vi "Receive-and-verify.vi"(8 "error in (no error)":errorcluster, 9 "Match exactly?":bool, 10 "Expected return string":string, 11 "SM1000-control in":refnum<class "MC-SM1000.lvclass">) -> (0 "error out":errorcluster, 1 "Verified?":bool, 2 "Return string":string, 3 "SM1000-control out":refnum<class "MC-SM1000.lvclass">)   [LabVIEW 2013, in "MaterialCharacterization.lvlib" / "MC-SM1000.lvclass"]
doc: "Verified if the return string contains at least the \nexpected string. Case insensitive."
uses:
  MC-SM1000.lvclass
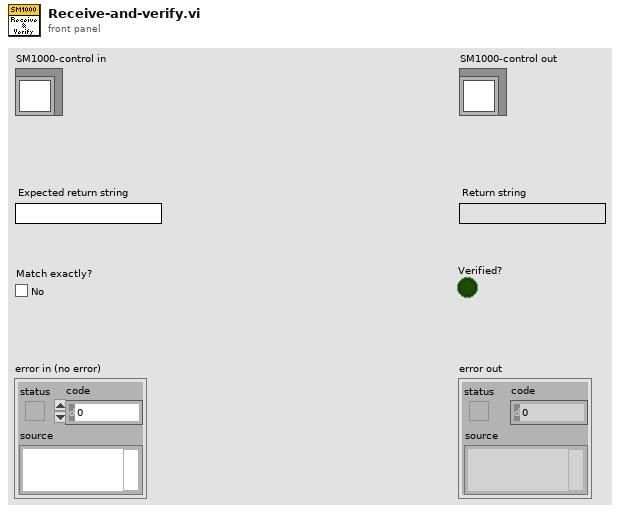
[diagram p1: front panel]
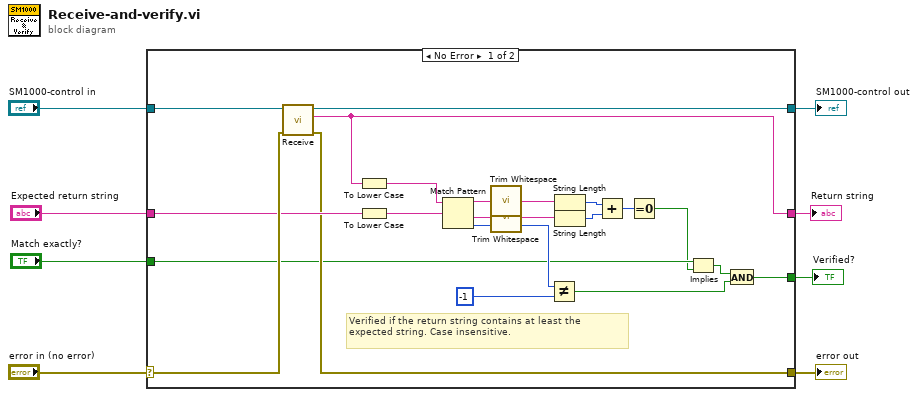
[diagram p0: block diagram]
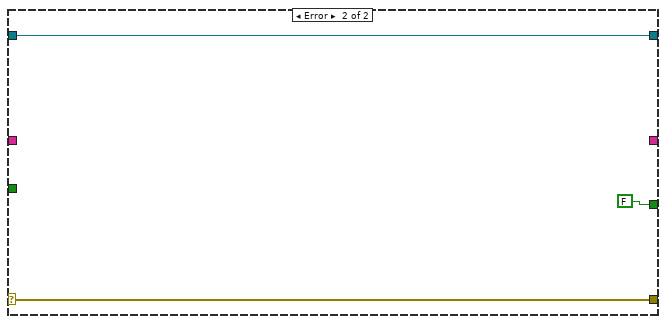
[diagram p2: hidden frame]
diagram:
  n1 = case shown="No Error" "error in (no error)" {
    selector: "error in (no error)" -> [w28 w33]
    tunnel: [w23 w33] -> w7
    tunnel: [w29 w32] -> w5
    tunnel: "SM1000-control in" -> [w30 w32]
    tunnel: [w24 _] -> w4
    tunnel: "Expected return string" -> [w27 _]
    tunnel: [w13 FALSE] -> w2
    tunnel: "Match exactly?" -> [w17 _]
    frame No Error {
      # "Verified if the return string contains at least the \nexpected string. Case insensitive."
      n2 = call "Receive.vi"("error in (no error)"=w28, "SM1000-control in"=w30) -> ("error out"=w23:errorcluster, "Return string"=w24:string, "SM1000-control out"=w29:refnum<class "MC-SM1000.lvclass">)  [unwired: 7 in]
      n3 = To Lower Case(string=w24) -> (all lower case string=w26:string)
      n4 = To Lower Case(string=w27) -> (all lower case string=w25:string)
      n5 = Match Pattern(string=w26, regular expression=w25) -> (before substring=w12:string, after substring=w11:string, offset past match=w21:i32)  [unwired: 1 in, 1 out]
      n6 = call <vilib>:"Trim Whitespace.vi"("string"=w12) -> ("trimmed string"=w9:string)  [unwired: 1 in]
      n7 = call <vilib>:"Trim Whitespace.vi"("string"=w11) -> ("trimmed string"=w10:string)  [unwired: 1 in]
      n8 = Not Equal?(x=w21, y=-1) -> (x != y?=w14:bool)
      n9 = String Length(string=w9) -> (length=w19:i32)
      n10 = String Length(string=w10) -> (length=w20:i32)
      n11 = Add(x=w19, y=w20) -> (x+y=w18:i32)
      n12 = Equal To 0?(x=w18) -> (x = 0?=w16:bool)
      n13 = Implies(1:w16, 2:w17) -> (0:w15:bool)
      n14 = And(x=w15, y=w14) -> (x .and. y?=w13:bool)
    }
    frame Error {
    }
  }
  "error out" <- w7
  "SM1000-control out" <- w5
  "Return string" <- w4
  "Verified?" <- w2
